vi "Yokogawa WT200 Series Time Integration.vi"(0 "VISA resource name":refnum<visa-resource-name>, 5 "Hour (0)":u32 max=10000, 7 "Minute (0)":u32 max=59 step=1, 9 "Second (0)":u32 max=59 step=1, 11 "error in (no error)":errorcluster) -> (4 "VISA resource name out":refnum<visa-resource-name>, 15 "error out":errorcluster)   [LabVIEW 2016]
doc: "This VI starts normal integration and waits until the end of the integration."
uses:
  Yokogawa WT200 Series.lvlib
panel:
  out "Second":i32 min=0 max=59 step=1
  out "sum":sgl
  out "Data":sgl[](array[numeric]) format="%^.3e"
  out "V Hz":sgl caption="Measure Value" format="%^.3e"
  out "Measure Value":sgl[](array[numeric]) format="%^.3e"
  # "© 2005 National Instruments.  ALL RIGHTS RESERVED."
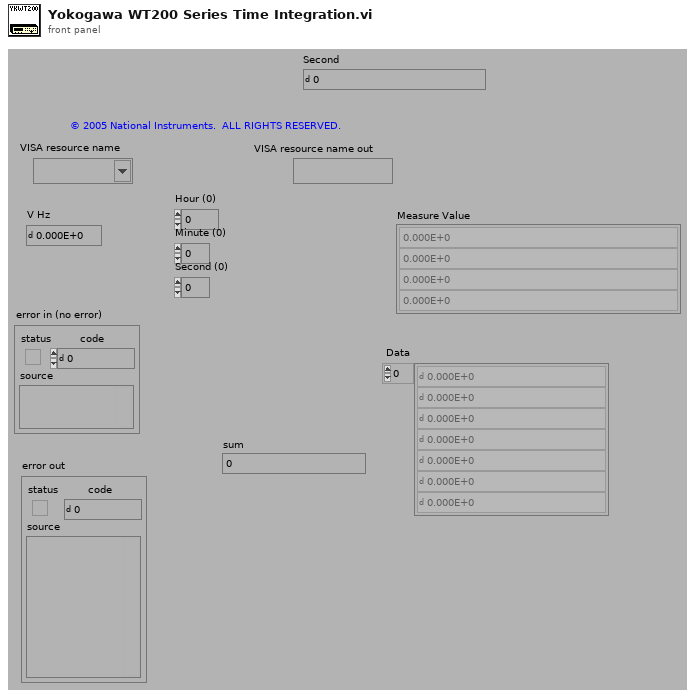
[diagram p1: front panel]
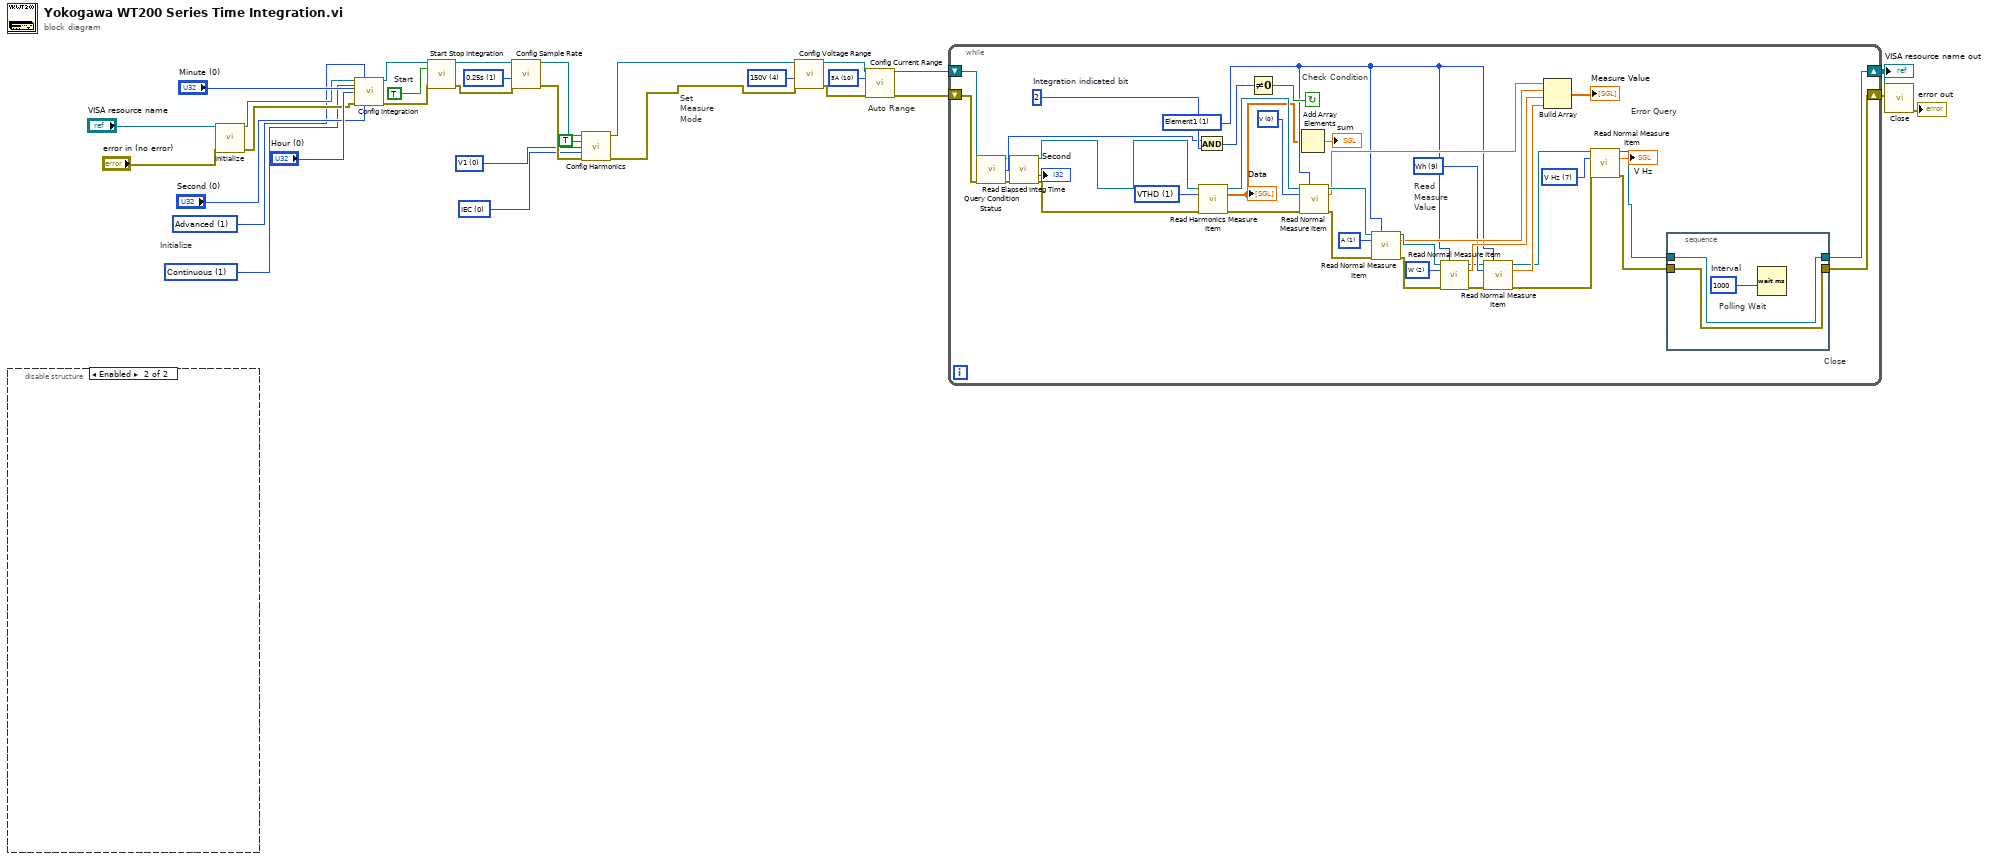
[diagram p0: block diagram]
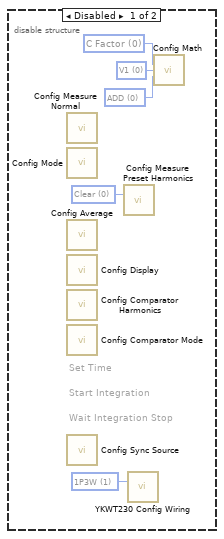
[diagram p2: hidden frame]
diagram:
  w4 = u16 0 items=["V1", "A1", "V2", "A2", "V3", "A3"] ("PLL source (0: V1)")
  w5 = u16 0 items=["IEC", "CSA"] ("THD (0: IEC)")
  w10 = u16 1 items=["0.1s", "0.25s", "0.5s", "1s", "2s", "5s"] ("Sample Rate (1: 0.25s)")
  w11 = u16 1 items=["Normal", "Continuous"] ("Integ Mode (0: Normal)")
  w17 = u16 10 items=["Auto", "5mA", "10mA", "20mA", "50mA", "100mA", "200mA", "0.5A", "1A", "2A", "5A", "10A", "20A", "50mV", "100mV", "200mV", "2.5V", "5V", "10V"] ("A Range (12: 20A)")
  w16 = u16 4 items=["Auto", "15V", "30V", "60V", "150V", "300V", "600V"] ("V Range (6: 600V)")
  w18 = u16 1 items=["Standard", "Advanced"] ("Integ Type (0: Standard)")
  w26 = TRUE  # Start
  # "Auto Range"
  # "Set \nMeasure \nMode"
  # "Initialize"
  n1 = disable-structure shown="Enabled" {
    frame Disabled {
      w32 = u16 0 items=["Clear", "V Pattern", "A Pattern", "W Pattern", "D Pattern", "All"] ("Preset Pattern (0: Clear)")
      w33 = u16 1 items=["", "1P3W", "3P3W", "3P4W", "3V3A"] ("Wiring (1: 1P3W)")
      w34 = u16 0 items=["ADD", "SUB", "MUL", "DIV", "DIVA", "DIVB"] ("Arithmetic (0: ADD)")
      w35 = u16 0 items=["V1", "A1", "V2", "A2", "V3", "A3"] ("C Factor (0: V)")
      w36 = u16 0 items=["C Factor", "Arithmetic", "Average", "Efficiency"] ("Math Type (0: Crest Factor)")
      # "Set Time"
      # "Start Integration"
      # "Wait Integration Stop"
      n2 = call "Config Measure Normal.vi"() -> ()  [unwired: 14 in, 2 out]
      n3 = call "Config Mode.vi"() -> ()  [unwired: 14 in, 2 out]
      n4 = call "Config Average.vi"() -> ()  [unwired: 14 in, 2 out]
      n5 = call "Config Display.vi"() -> ()  [unwired: 14 in, 2 out]
      n6 = call "Config Comparator Harmonics.vi"() -> ()  [unwired: 14 in, 2 out]
      n7 = call "Config Comparator Mode.vi"() -> ()  [unwired: 14 in, 2 out]
      n8 = call "Config Sync Source.vi"() -> ()  [unwired: 14 in, 2 out]
      n9 = call "Config Measure Preset Harmonics.vi"("Preset Pattern (0: Clear)"=w32) -> ()  [unwired: 13 in, 2 out]
      n10 = call "YKWT230 Config Wiring.vi"("Wiring (1: 1P3W)"=w33) -> ()  [unwired: 13 in, 2 out]
      n11 = call "Config Math.vi"("Math Type (0: Crest Factor)"=w36, "C Factor (0: V)"=w35, "Arithmetic (0: ADD)"=w34) -> ()  [unwired: 11 in, 2 out]
    }
    frame Enabled {
    }
  }
  n12 = call "Initialize.vi"("VISA resource name"="VISA resource name", "error in (no error)"="error in (no error)") -> ("VISA resource name out"=w25:refnum<visa-resource-name>, "error out"=w24:errorcluster)  [unwired: 11 in, 1 out]
  n13 = call "Config Integration.vi"("VISA resource name"=w25, "Integ Type (0: Standard)"=w18, "Integ Mode (0: Normal)"=w11, "Hour (0)"="Hour (0)", "Minute (0)"="Minute (0)", "error in (no error)"=w24, "Second (0)"="Second (0)") -> ("VISA resource name out"=w30:refnum<visa-resource-name>, "error out"=w31:errorcluster)  [unwired: 7 in]
  n14 = call "Start Stop Integration.vi"("VISA resource name"=w30, "Start/Stop (F: Stop)"=w26, "error in (no error)"=w31) -> ("VISA resource name out"=w8:refnum<visa-resource-name>, "error out"=w9:errorcluster)  [unwired: 11 in]
  n15 = call "Config Sample Rate.vi"("VISA resource name"=w8, "Sample Rate (1: 0.25s)"=w10, "error in (no error)"=w9) -> ("VISA resource name out"=w7:refnum<visa-resource-name>, "error out"=w6:errorcluster)  [unwired: 11 in]
  n16 = call "Config Harmonics.vi"("VISA resource name"=w7, "Harmonic Mode (F: OFF)"=TRUE, "PLL source (0: V1)"=w4, "THD (0: IEC)"=w5, "error in (no error)"=w6) -> ("VISA resource name out"=w2:refnum<visa-resource-name>, "error out"=w1:errorcluster)  [unwired: 9 in]
  n17 = call "Config Voltage Range.vi"("VISA resource name"=w2, "V Range (6: 600V)"=w16, "error in (no error)"=w1) -> ("VISA resource name out"=w15:refnum<visa-resource-name>, "error out"=w14:errorcluster)  [unwired: 11 in]
  n18 = call "Config Current Range.vi"("VISA resource name"=w15, "A Range (12: 20A)"=w17, "error in (no error)"=w14) -> ("VISA resource name out"=w12:refnum<visa-resource-name>, "error out"=w13:errorcluster)  [unwired: 11 in]
  n19 = while {
    shift-left: w12 -> [w72]
    shift-right: [w70] -> w20
    shift-left: w13 -> [w73]
    shift-right: [w71] -> w21
    stop <- w75 continue-if-true
    w46 = u16 1 items=["Sync", "VTHD", "V", "VCON", "ATHD", "A", "ACON", "PF", "W", "WCON", "Vdeg", "Adeg"] ("Harmonics Item (2: V)")
    w50 = u16 7 items=["V", "A", "W", "VA", "var", "PF", "deg", "V Hz", "A Hz", "Wh", "Wh+", "Wh-", "Ah", "Ah+", "Ah-", "Vpk", "Apk", "Math"] ("Measure Item (0: V)")
    w56 = u16 9 items=["V", "A", "W", "VA", "var", "PF", "deg", "V Hz", "A Hz", "Wh", "Wh+", "Wh-", "Ah", "Ah+", "Ah-", "Vpk", "Apk", "Math"] ("Measure Item (0: V)")
    w54 = u16 1 items=["", "Element1", "Element2", "Element3", "Sigma"] ("Element (1: Element 1)")
    w59 = u16 0 items=["V", "A", "W", "VA", "var", "PF", "deg", "V Hz", "A Hz", "Wh", "Wh+", "Wh-", "Ah", "Ah+", "Ah-", "Vpk", "Apk", "Math"] ("Measure Item (0: V)")
    w60 = u16 2 items=["V", "A", "W", "VA", "var", "PF", "deg", "V Hz", "A Hz", "Wh", "Wh+", "Wh-", "Ah", "Ah+", "Ah-", "Vpk", "Apk", "Math"] ("Measure Item (0: V)")
    w61 = u16 1 items=["V", "A", "W", "VA", "var", "PF", "deg", "V Hz", "A Hz", "Wh", "Wh+", "Wh-", "Ah", "Ah+", "Ah-", "Vpk", "Apk", "Math"] ("Measure Item (0: V)")
    w76 = u16 2  # Integration indicated bit
    # "Error Query"
    # "Close"
    # "Read\nMeasure\nValue"
    # "Check Condition"
    n20 = call "Query Condition Status.vi"("VISA resource name"=w72, "error in (no error)"=w73) -> ("VISA resource name out"=w43:refnum<visa-resource-name>, "Condition"=w69:u16, "error out"=w42:errorcluster)  [unwired: 11 in]
    n21 = call "Read Elapsed Integ Time.vi"("VISA resource name"=w43, "error in (no error)"=w42) -> ("VISA resource name out"=w40:refnum<visa-resource-name>, "Second"=→"Second":i32, "error out"=w39:errorcluster)  [unwired: 9 in, 2 out]
    n22 = And(x=w69, y=w76) -> (x .and. y?=w74:u16)
    n23 = call "Read Harmonics Measure Item.vi"("VISA resource name"=w40, "Harmonics Item (2: V)"=w46, "error in (no error)"=w39) -> ("VISA resource name out"=w48:refnum<visa-resource-name>, "Data"=w45:sgl[], "error out"=w47:errorcluster)  [unwired: 10 in]
    "Data" <- w45
    n24 = Not Equal To 0?(x=w74) -> (x != 0?=w75:bool)
    n25 = Add Array Elements(numeric array=w45) -> (sum=→"sum":sgl)
    n26 = call "Read Normal Measure Item.vi"("VISA resource name"=w48, "Element (1: Element 1)"=w54, "Measure Item (0: V)"=w59, "error in (no error)"=w47) -> ("VISA resource name out"=w66:refnum<visa-resource-name>, "Measure Value"=w62:sgl, "error out"=w68:errorcluster)  [unwired: 9 in]
    n27 = call "Read Normal Measure Item.vi"("VISA resource name"=w66, "Element (1: Element 1)"=w54, "Measure Item (0: V)"=w61, "error in (no error)"=w68) -> ("VISA resource name out"=w65:refnum<visa-resource-name>, "Measure Value"=w63:sgl, "error out"=w67:errorcluster)  [unwired: 9 in]
    n28 = call "Read Normal Measure Item.vi"("VISA resource name"=w65, "Element (1: Element 1)"=w54, "Measure Item (0: V)"=w60, "error in (no error)"=w67) -> ("VISA resource name out"=w55:refnum<visa-resource-name>, "Measure Value"=w64:sgl, "error out"=w57:errorcluster)  [unwired: 9 in]
    n29 = call "Read Normal Measure Item.vi"("VISA resource name"=w55, "Element (1: Element 1)"=w54, "Measure Item (0: V)"=w56, "error in (no error)"=w57) -> ("VISA resource name out"=w51:refnum<visa-resource-name>, "Measure Value"=w53:sgl, "error out"=w52:errorcluster)  [unwired: 9 in]
    n30 = Build Array(w62, w63, w64, w53) -> (→"Measure Value":sgl[])
    n31 = call "Read Normal Measure Item.vi"("VISA resource name"=w51, "Measure Item (0: V)"=w50, "error in (no error)"=w52) -> ("VISA resource name out"=w37:refnum<visa-resource-name>, "Measure Value"=→"V Hz":sgl, "error out"=w38:errorcluster)  [unwired: 10 in]
    n32 = stacked-sequence {
      tunnel: w38 -> [w78]
      tunnel: [w78] -> w71
      tunnel: w37 -> [w77]
      tunnel: [w77] -> w70
      frame #0 {
        w79 = u32 1000  # Interval
        # "Polling Wait"
        n33 = Wait (ms)(milliseconds to wait=w79) -> ()  [unwired: 1 out]
      }
    }
  }
  "VISA resource name out" <- w20
  n34 = call "Close.vi"("VISA resource name"=w20, "error in (no error)"=w21) -> ("error out"=→"error out":errorcluster)  [unwired: 13 in]
